vi "Calculate - Class.vi"() -> ()   [LabVIEW 2013]
uses:
  Operators/Addition/Addition.lvclass
  Operators/Divide/Divide.lvclass
  Operators/Multiply/Multiply.lvclass
  Operators/Subtraction/Subtraction.lvclass
  Calculate/Calculate/Calculate.lvclass
panel:
  in  "btnDivide":bool
  in  "btnMultiply":bool
  in  "btnSubtract":bool
  in  "btnStop":bool
  in  "btnAdd":bool
  out "Result":dbl
  in  "Operand 2":dbl
  in  "Operand 1":dbl
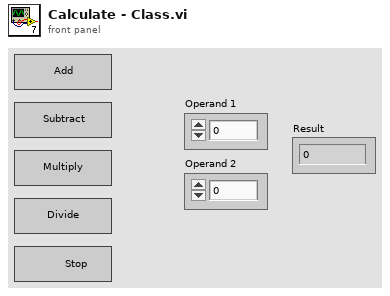
[diagram p1: front panel]
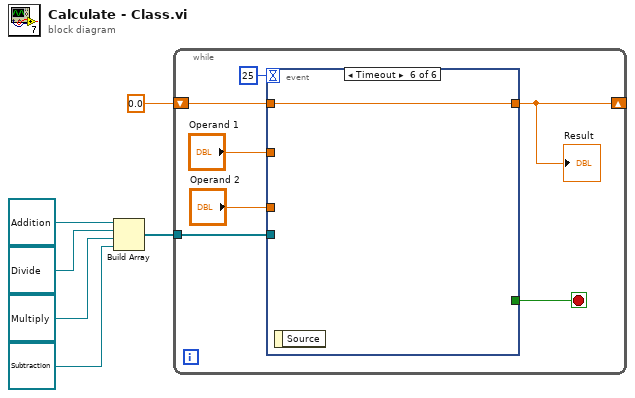
[diagram p0: block diagram]
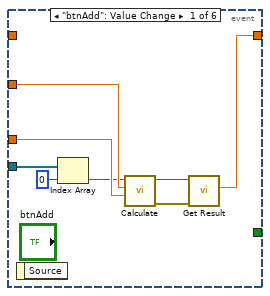
[diagram p2: hidden frame]
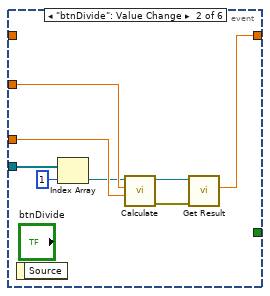
[diagram p3: hidden frame]
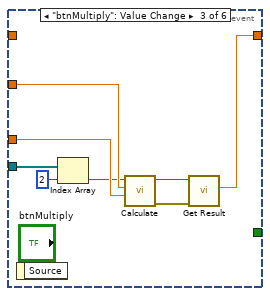
[diagram p4: hidden frame]
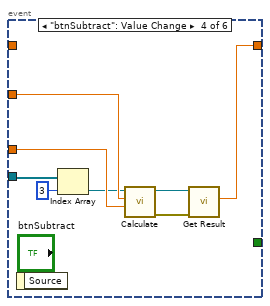
[diagram p5: hidden frame]
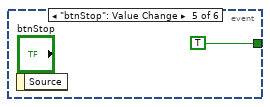
[diagram p6: hidden frame]
diagram:
  n1 = Build Array(refnum<class "Addition.lvclass"> refnum ("Operators.lvlib:Addition.lvclass"), refnum<class "Divide.lvclass"> refnum ("Operators.lvlib:Divide.lvclass"), refnum<class "Multiply.lvclass"> refnum ("Operators.lvlib:Multiply.lvclass"), refnum<class "Subtraction.lvclass"> refnum ("Operators.lvlib:Subtraction.lvclass")) -> (w2:refnum<class "Calculate.lvclass">[])
  n2 = while {
    tunnel: w2 -> [w11]
    shift-right: [w9] -> _
    shift-left: 0.0 ("Result") -> [w7]
    stop <- w10 stop-if-true
    n3 = event shown="[5] Timeout" {
      selector: _ -> [_ _ _ _ _ _]
      dyn-events: _ -> [_ _ _ _ _ _]
      timeout: 25 -> [_ _ _ _ _ _]
      tunnel: "Operand 1" -> [w21 w29 w37 w45 _ _]
      tunnel: "Operand 2" -> [w20 w28 w36 w44 _ _]
      tunnel: w11 -> [w18 w26 w34 w42 _ _]
      tunnel: [w14 w22 w30 w38 _ w47] -> w9
      tunnel: [_ _ _ _ TRUE _] -> w10
      tunnel: w7 -> [_ _ _ _ _ w47]
      event "btnAdd": Value Change {
        n4 = event-data() -> ()  [unwired: 1 in, 1 out]
        n5 = Index Array(array=w18, index=0) -> (element=w17:refnum<class "Calculate.lvclass">)
        n6 = call-dynamic "Calculate.vi"("Operand 2"=w20, "Operand 1"=w21, "Calculate in"=w17) -> ("error out"=w15:errorcluster, "Calculate out"=w19:refnum<class "Calculate.lvclass">)  [unwired: 7 in]
        n7 = call-dynamic "Get Result.vi"("error in (no error)"=w15, "Calculate in"=w19) -> ("Result"=w14:dbl)  [unwired: 7 in, 2 out]
      }
      event "btnDivide": Value Change {
        n8 = event-data() -> ()  [unwired: 1 in, 1 out]
        n9 = Index Array(array=w26, index=1) -> (element=w25:refnum<class "Calculate.lvclass">)
        n10 = call-dynamic "Calculate.vi"("Operand 2"=w28, "Operand 1"=w29, "Calculate in"=w25) -> ("error out"=w23:errorcluster, "Calculate out"=w27:refnum<class "Calculate.lvclass">)  [unwired: 7 in]
        n11 = call-dynamic "Get Result.vi"("error in (no error)"=w23, "Calculate in"=w27) -> ("Result"=w22:dbl)  [unwired: 7 in, 2 out]
      }
      event "btnMultiply": Value Change {
        n12 = event-data() -> ()  [unwired: 1 in, 1 out]
        n13 = Index Array(array=w34, index=2) -> (element=w33:refnum<class "Calculate.lvclass">)
        n14 = call-dynamic "Calculate.vi"("Operand 2"=w36, "Operand 1"=w37, "Calculate in"=w33) -> ("error out"=w31:errorcluster, "Calculate out"=w35:refnum<class "Calculate.lvclass">)  [unwired: 7 in]
        n15 = call-dynamic "Get Result.vi"("error in (no error)"=w31, "Calculate in"=w35) -> ("Result"=w30:dbl)  [unwired: 7 in, 2 out]
      }
      event "btnSubtract": Value Change {
        n16 = event-data() -> ()  [unwired: 1 in, 1 out]
        n17 = Index Array(array=w42, index=3) -> (element=w41:refnum<class "Calculate.lvclass">)
        n18 = call-dynamic "Calculate.vi"("Operand 2"=w44, "Operand 1"=w45, "Calculate in"=w41) -> ("error out"=w39:errorcluster, "Calculate out"=w43:refnum<class "Calculate.lvclass">)  [unwired: 7 in]
        n19 = call-dynamic "Get Result.vi"("error in (no error)"=w39, "Calculate in"=w43) -> ("Result"=w38:dbl)  [unwired: 7 in, 2 out]
      }
      event "btnStop": Value Change {
        n20 = event-data() -> ()  [unwired: 1 in, 1 out]
      }
      event Timeout {
        n21 = event-data() -> ()  [unwired: 1 in, 1 out]
      }
    }
    "Result" <- w9
  }
